vi "ConnectToRobot.vi"(0 "error in":errorcluster, 1 "address":string, 2 "Telnet enable":bool, 3 "Telnet KCL password":string, 4 "SNPX enable":bool, 5 "FTP enable":bool, 6 "FTP user":string, 7 "FTP password":string, 9 "CGTP enable":bool, 11 "HTTP login":string, 13 "HTTP password":string) -> (20 "error out":errorcluster, 21 "robot":refnum<k24>, 24 "Telnet":refnum<k24>, 25 "Ftp":refnum<k24>, 26 "Snpx":refnum<k24>, 27 "Cgtp":refnum<k24>)   [LabVIEW 2024, in "UnderAutomation.Fanuc.lvlib"]
uses:
  UnderAutomation.Fanuc.lvlib
  C:/Users/fg/Documents/Fanuc.vi/LabVIEW_2024/UnderAutomation.Fanuc/lib/UnderAutomation.Fanuc.dll
  lib/UnderAutomation.Fanuc.dll
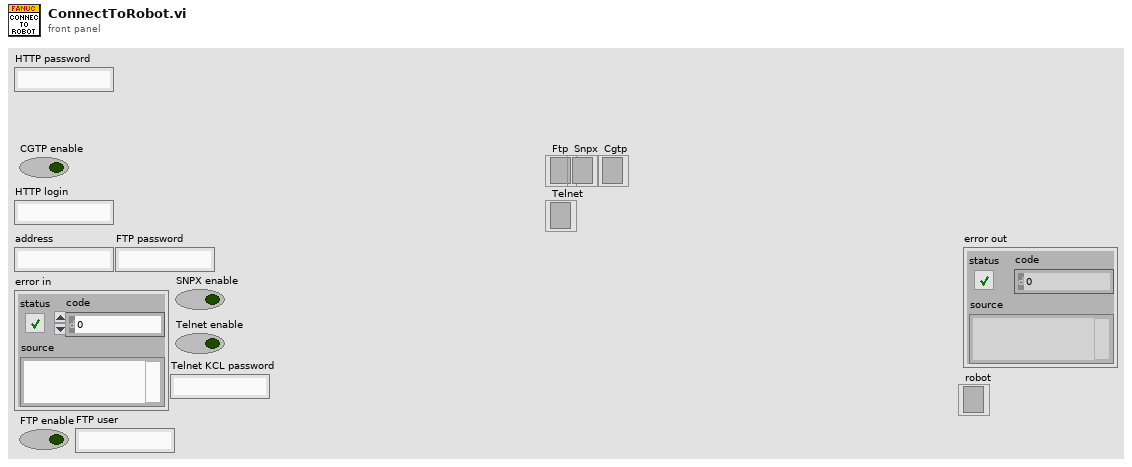
[diagram p1: front panel]
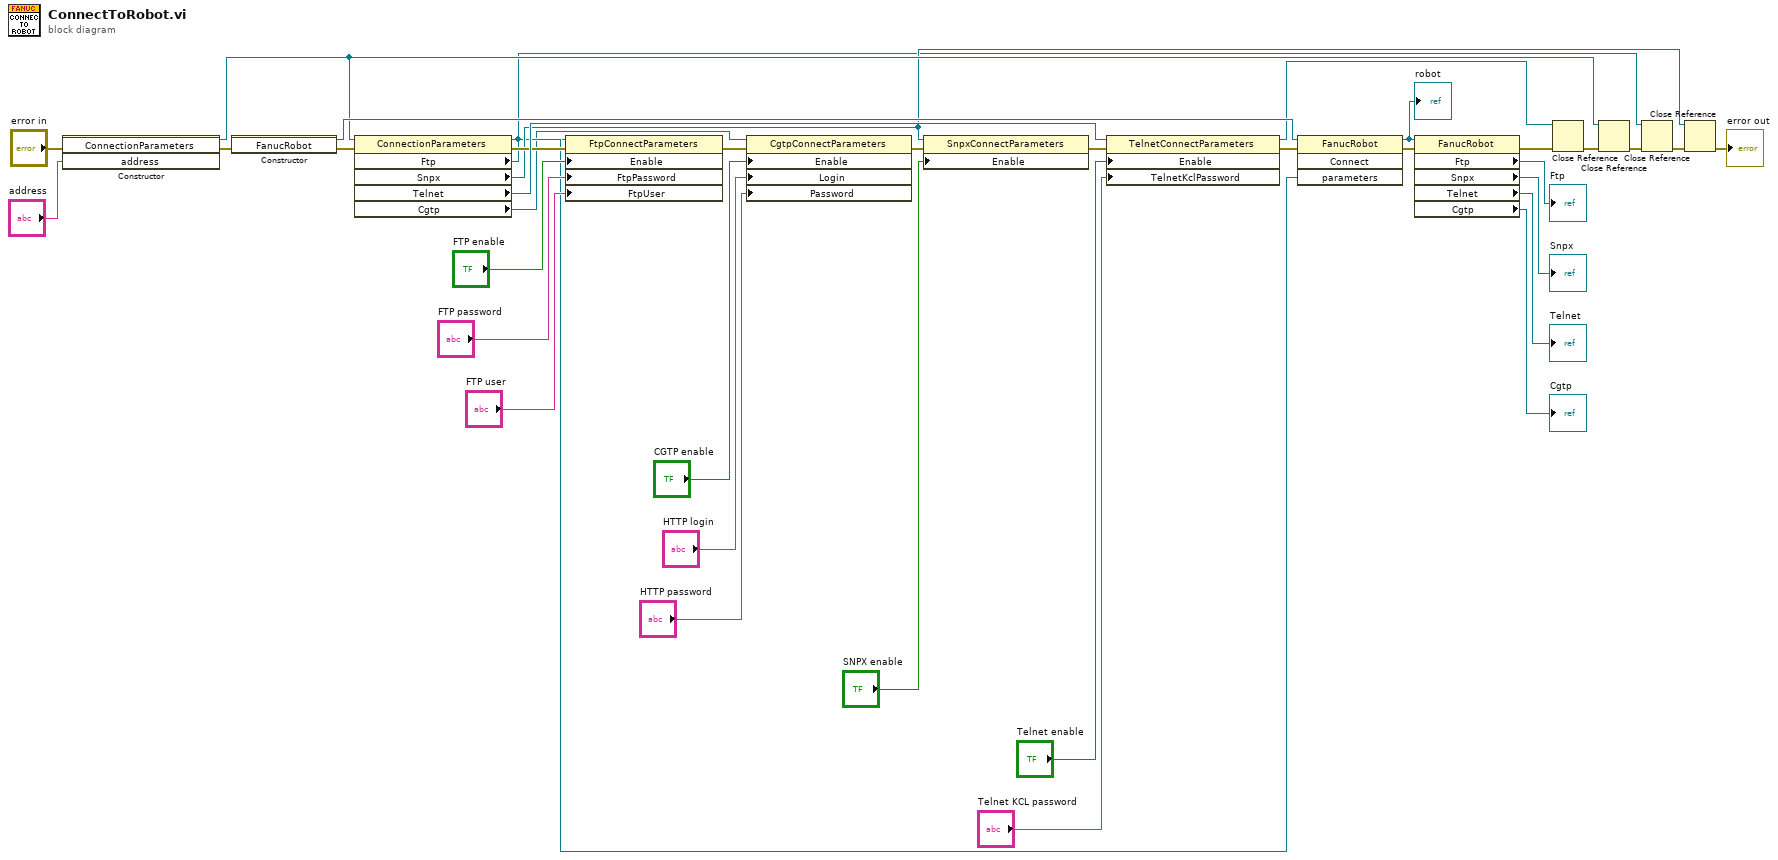
[diagram p0: block diagram]
diagram:
  n1 = constructor class="ConnectionParameters"(error in="error in", "address"="address") -> (reference out=w14:refnum<k24>, error out=w36:errorcluster)  [unwired: 2 in, 2 out]
  n2 = constructor class="FanucRobot"(error in=w36) -> (reference out=w37:refnum<k24>, error out=w30:errorcluster)  [unwired: 2 in, 1 out]
  n3 = property class="ConnectionParameters"(reference=w14, error in=w30) -> (reference out=w12:refnum<k24>, error out=w32:errorcluster, "Ftp"=w11:refnum<k24>, "Snpx"=w13:refnum<k24>, "Telnet"=w34:refnum<k24>, "Cgtp"=w6:refnum<k24>)
  n4 = property class="FtpConnectParameters"(reference=w11, error in=w32, "Enable"="FTP enable", "FtpPassword"="FTP password", "FtpUser"="FTP user") -> (error out=w5:errorcluster)  [unwired: 1 out]
  n5 = property class="CgtpConnectParameters"(reference=w6, error in=w5, "Enable"="CGTP enable", "Login"="HTTP login", "Password"="HTTP password") -> (error out=w4:errorcluster)  [unwired: 1 out]
  n6 = property class="SnpxConnectParameters"(reference=w13, error in=w4, "Enable"="SNPX enable") -> (error out=w31:errorcluster)  [unwired: 1 out]
  n7 = property class="TelnetConnectParameters"(reference=w34, error in=w31, "Enable"="Telnet enable", "TelnetKclPassword"="Telnet KCL password") -> (reference out=w17:refnum<k24>, error out=w29:errorcluster)
  n8 = invoke class="FanucRobot" method="Connect"(reference=w37, error in=w29, "parameters"=w12) -> (reference out=w22:refnum<k24>, error out=w21:errorcluster)  [unwired: 1 in, 2 out]
  "robot" <- w22
  n9 = property class="FanucRobot"(reference=w22, error in=w21) -> (error out=w16:errorcluster, "Ftp"=→"Ftp":refnum<k24>, "Snpx"=→"Snpx":refnum<k24>, "Telnet"=→"Telnet":refnum<k24>, "Cgtp"=→"Cgtp":refnum<k24>)  [unwired: 1 out]
  n10 = Close Reference(reference=w17, error in (no error)=w16) -> (error out=w15:errorcluster)
  n11 = Close Reference(reference=w14, error in (no error)=w15) -> (error out=w10:errorcluster)
  n12 = Close Reference(reference=w11, error in (no error)=w10) -> (error out=w9:errorcluster)
  n13 = Close Reference(reference=w13, error in (no error)=w9) -> (error out=→"error out":errorcluster)
